vi "QueueControl.vi"(10 "Enum":T1(ring), 11 "RefIn":refnum<vi>) -> ()   [LabVIEW 2019]
uses:
  QueueControl.ctl
panel:
  # "Queue :"
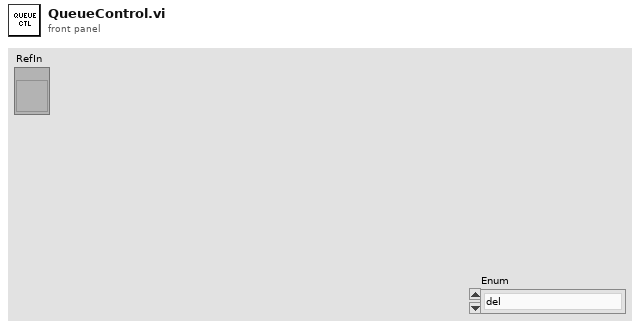
[diagram p1: front panel]
types:
  T1 = enum16{"del", "update", "down", "up", "bot", "top"}
  T2 = typedef "QueueControl.ctl" = cluster{"QueueFromServer":i32, "First Queue":string, "Add To Queue:":string, "Up":bool, "Down":bool, "Del":bool, "Front":bool, "Back":bool, "Next":bool, "Combo Box":string}
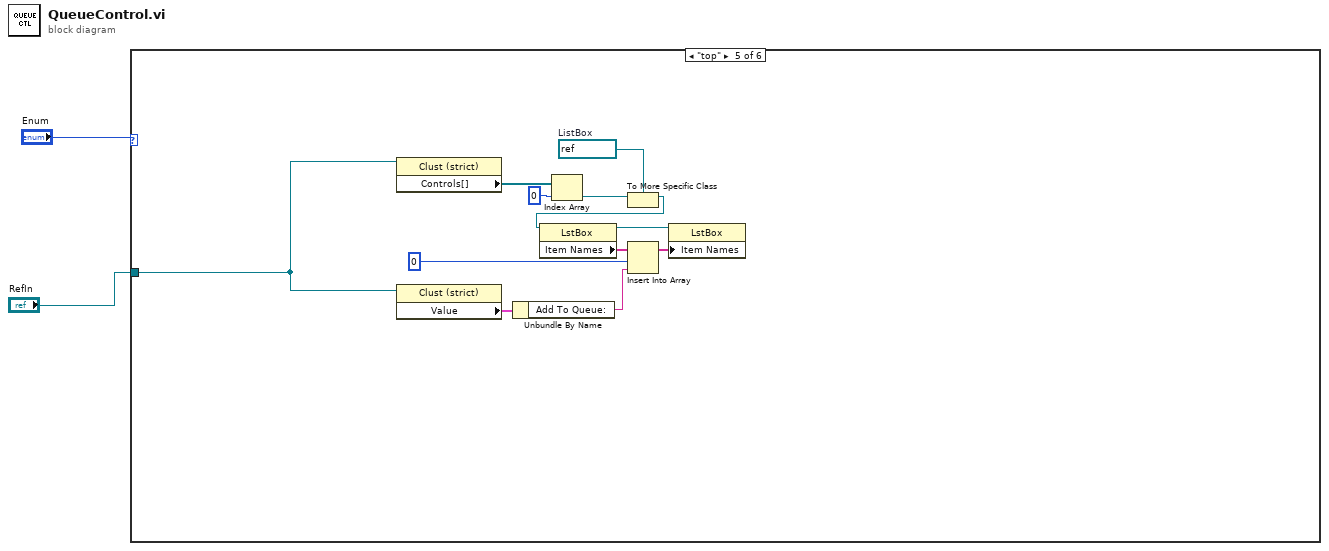
[diagram p0: block diagram]
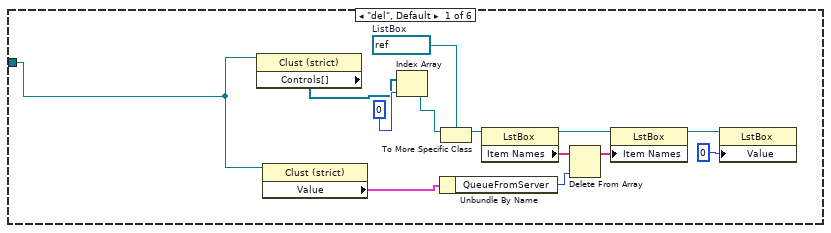
[diagram p2: hidden frame]
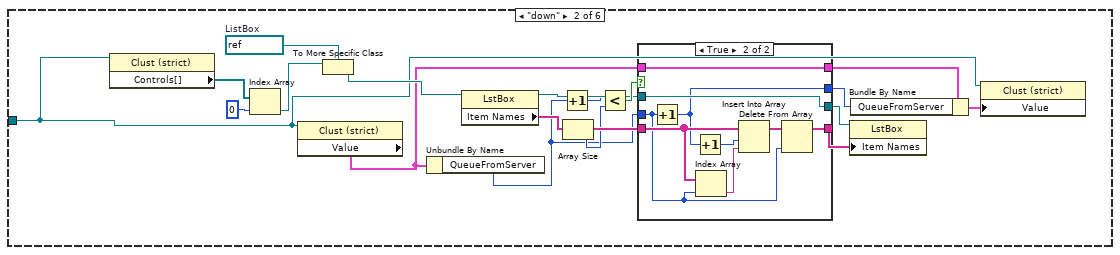
[diagram p3: hidden frame]
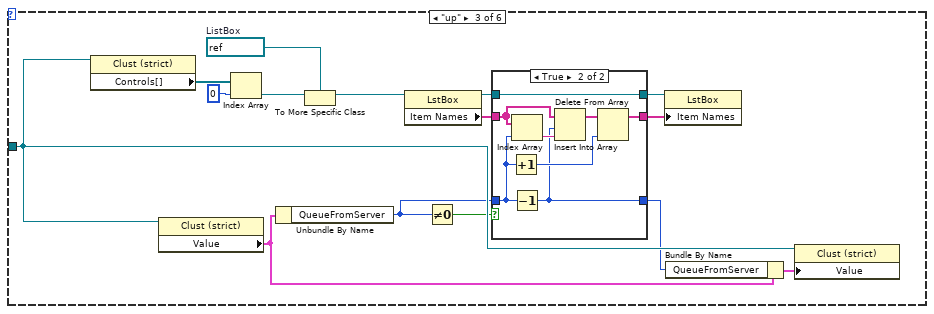
[diagram p5: hidden frame]
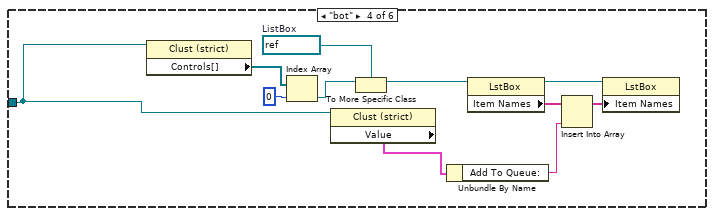
[diagram p7: hidden frame]
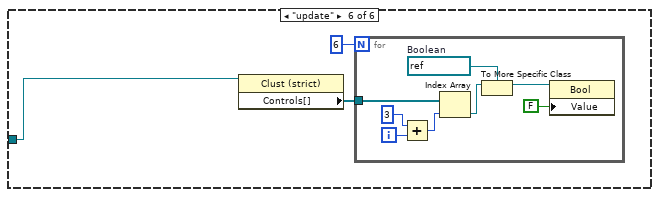
[diagram p8: hidden frame]
diagram:
  n1 = case shown="\"top\"" "Enum" {
    tunnel: "RefIn" -> [w3 w16 w55 w73 w86 w96]
    frame "del", Default {
      w6 = refnum<vi> refnum  # ListBox
      n2 = property class="Clust (strict)"(reference=w3) -> ("Controls[]"=w7:refnum<vi>[])  [unwired: 1 in, 2 out]
      n3 = property class="Clust (strict)"(reference=w3) -> ("Value"=w4:T2)  [unwired: 1 in, 2 out]
      n4 = Index Array(array=w7, index=0) -> (element=w5:refnum<vi>)
      n5 = Unbundle By Name(w4) -> ("QueueFromServer"=w11:i32)
      n6 = To More Specific Class(target class=w6, reference=w5) -> (specific class reference=w9:refnum<vi>)  [unwired: 1 in, 1 out]
      n7 = property class="LstBox"(reference=w9) -> (reference out=w13:refnum<vi>, "Item Names"=w10:string[])  [unwired: 1 in, 1 out]
      n8 = Delete From Array(array=w10, index=w11) -> (array with subset deleted=w12:string[])  [unwired: 1 in, 1 out]
      n9 = property class="LstBox"(reference=w13, "Item Names"=w12) -> (reference out=w14:refnum<vi>)  [unwired: 1 in, 1 out]
      n10 = property class="LstBox"(reference=w14, "Value"=0) -> ()  [unwired: 1 in, 2 out]
    }
    frame "down" {
      w31 = refnum<vi> refnum  # ListBox
      n11 = property class="Clust (strict)"(reference=w16) -> ("Controls[]"=w30:refnum<vi>[])  [unwired: 1 in, 2 out]
      n12 = Index Array(array=w30, index=0) -> (element=w32:refnum<vi>)
      n13 = property class="Clust (strict)"(reference=w16) -> ("Value"=w26:T2)  [unwired: 1 in, 2 out]
      n14 = To More Specific Class(target class=w31, reference=w32) -> (specific class reference=w29:refnum<vi>)  [unwired: 1 in, 1 out]
      n15 = Unbundle By Name(w26) -> ("QueueFromServer"=w17:i32)
      n16 = property on="Property Node" class="LstBox"(reference=w29) -> (reference out=w22:refnum<vi>, "Item Names"=w20:string[])  [unwired: 1 in, 1 out]
      n17 = Increment(x=w17) -> (x+1=w18:i32)
      n18 = Array Size(array=w20) -> (size(s)=w19:i32)
      n19 = Less?(x=w18, y=w19) -> (x < y?=w28:bool)
      n20 = case shown="True" w28 {
        tunnel: w17 -> [w35 w39]
        tunnel: w20 -> [w36 w44]
        tunnel: [w35 w38] -> w27
        tunnel: w26 -> [w34 w43]
        tunnel: [w34 w43] -> w25
        tunnel: [w36 w42] -> w23
        tunnel: w22 -> [w37 w41]
        tunnel: [w37 w41] -> w21
        frame False {
        }
        frame True {
          n21 = Increment(x=w39) -> (x+1=w38:i32)
          n22 = Increment(x=w38) -> (x+1=w40:i32)
          n23 = Index Array(array=w44, index=w39) -> (element=w46:string)
          n24 = Insert Into Array(array=w44, index=w40, new element=w46) -> (w45:string[])
          n25 = Delete From Array(array=w45, index=w39) -> (array with subset deleted=w42:string[])  [unwired: 1 in, 1 out]
        }
      }
      n26 = property on="Property Node" class="LstBox"(reference=w21, "Item Names"=w23) -> ()  [unwired: 1 in, 2 out]
      n27 = Bundle By Name(cluster=w25, "QueueFromServer"=w27) -> (w24:T2)
      n28 = property class="Clust (strict)"(reference=w16, "Value"=w24) -> ()  [unwired: 1 in, 2 out]
    }
    frame "up" {
      w59 = refnum<vi> refnum  # ListBox
      n29 = property class="Clust (strict)"(reference=w55) -> ("Controls[]"=w60:refnum<vi>[])  [unwired: 1 in, 2 out]
      n30 = property class="Clust (strict)"(reference=w55) -> ("Value"=w56:T2)  [unwired: 1 in, 2 out]
      n31 = Index Array(array=w60, index=0) -> (element=w58:refnum<vi>)
      n32 = Unbundle By Name(w56) -> ("QueueFromServer"=w52:i32)
      n33 = To More Specific Class(target class=w59, reference=w58) -> (specific class reference=w61:refnum<vi>)  [unwired: 1 in, 1 out]
      n34 = property on="Property Node" class="LstBox"(reference=w61) -> (reference out=w48:refnum<vi>, "Item Names"=w53:string[])  [unwired: 1 in, 1 out]
      n35 = Not Equal To 0?(x=w52) -> (x != 0?=w51:bool)
      n36 = case shown="True" w51 {
        tunnel: w53 -> [w63 w69]
        tunnel: w52 -> [w62 w68]
        tunnel: [w62 w67] -> w50
        tunnel: [w63 w66] -> w49
        tunnel: w48 -> [w64 w65]
        tunnel: [w64 w65] -> w47
        frame False {
        }
        frame True {
          n37 = Increment(x=w68) -> (x+1=w72:i32)
          n38 = Index Array(array=w69, index=w68) -> (element=w70:string)
          n39 = Decrement(x=w68) -> (x-1=w67:i32)
          n40 = Insert Into Array(array=w69, index=w67, new element=w70) -> (w71:string[])
          n41 = Delete From Array(array=w71, index=w72) -> (array with subset deleted=w66:string[])  [unwired: 1 in, 1 out]
        }
      }
      n42 = property on="Property Node" class="LstBox"(reference=w47, "Item Names"=w49) -> ()  [unwired: 1 in, 2 out]
      n43 = Bundle By Name(cluster=w56, "QueueFromServer"=w50) -> (w54:T2)
      n44 = property class="Clust (strict)"(reference=w55, "Value"=w54) -> ()  [unwired: 1 in, 2 out]
    }
    frame "bot" {
      w77 = refnum<vi> refnum  # ListBox
      n45 = property on="Property Node" class="Clust (strict)"(reference=w73) -> ("Controls[]"=w74:refnum<vi>[])  [unwired: 1 in, 2 out]
      n46 = Index Array(array=w74, index=0) -> (element=w76:refnum<vi>)
      n47 = property class="Clust (strict)"(reference=w73) -> ("Value"=w79:T2)  [unwired: 1 in, 2 out]
      n48 = To More Specific Class(target class=w77, reference=w76) -> (specific class reference=w83:refnum<vi>)  [unwired: 1 in, 1 out]
      n49 = Unbundle By Name(w79) -> ("Add To Queue:"=w80:string)
      n50 = property on="Property Node" class="LstBox"(reference=w83) -> (reference out=w81:refnum<vi>, "Item Names"=w78:string[])  [unwired: 1 in, 1 out]
      n51 = Insert Into Array(array=w78, new element=w80) -> (w82:string[])  [unwired: 1 in]
      n52 = property on="Property Node" class="LstBox"(reference=w81, "Item Names"=w82) -> ()  [unwired: 1 in, 2 out]
    }
    frame "top" {
      w92 = refnum<vi> refnum  # ListBox
      n53 = property on="Property Node" class="Clust (strict)"(reference=w86) -> ("Controls[]"=w95:refnum<vi>[])  [unwired: 1 in, 2 out]
      n54 = property class="Clust (strict)"(reference=w86) -> ("Value"=w85:T2)  [unwired: 1 in, 2 out]
      n55 = Unbundle By Name(w85) -> ("Add To Queue:"=w90:string)
      n56 = Index Array(array=w95, index=0) -> (element=w93:refnum<vi>)
      n57 = To More Specific Class(target class=w92, reference=w93) -> (specific class reference=w84:refnum<vi>)  [unwired: 1 in, 1 out]
      n58 = property on="Property Node" class="LstBox"(reference=w84) -> (reference out=w89:refnum<vi>, "Item Names"=w91:string[])  [unwired: 1 in, 1 out]
      n59 = Insert Into Array(array=w91, index=0, new element=w90) -> (w88:string[])
      n60 = property on="Property Node" class="LstBox"(reference=w89, "Item Names"=w88) -> ()  [unwired: 1 in, 2 out]
    }
    frame "update" {
      n61 = property class="Clust (strict)"(reference=w96) -> ("Controls[]"=w97:refnum<vi>[])  [unwired: 1 in, 2 out]
      n62 = for {
        N: 6 -> [_]
        tunnel: w97 -> [w103]
        i -> [w106]
        w100 = refnum<vi> refnum  # Boolean
        n63 = Add(x=3, y=w106) -> (x+y=w104:i32)
        n64 = Index Array(array=w103, index=w104) -> (element=w102:refnum<vi>)
        n65 = To More Specific Class(target class=w100, reference=w102) -> (specific class reference=w101:refnum<vi>)  [unwired: 1 in, 1 out]
        n66 = property class="Bool"(reference=w101, "Value"=FALSE) -> ()  [unwired: 1 in, 2 out]
      }
    }
  }
